vi "SPI_Project.vi"() -> ()   [LabVIEW 2019]
uses:
  <vilib>/rvi/eio/common/nirviEmuTemplateMethod_errors.vi
  <vilib>/eio/EIONode/EIONode.xnode
  <vilib>/eio/EIOMethodNode/EIOMethodNode.xnode
panel:
  out "Device":u32
  in  "Dummy":u8 format="%b"
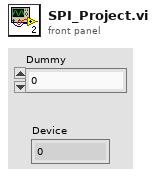
[diagram p1: front panel]
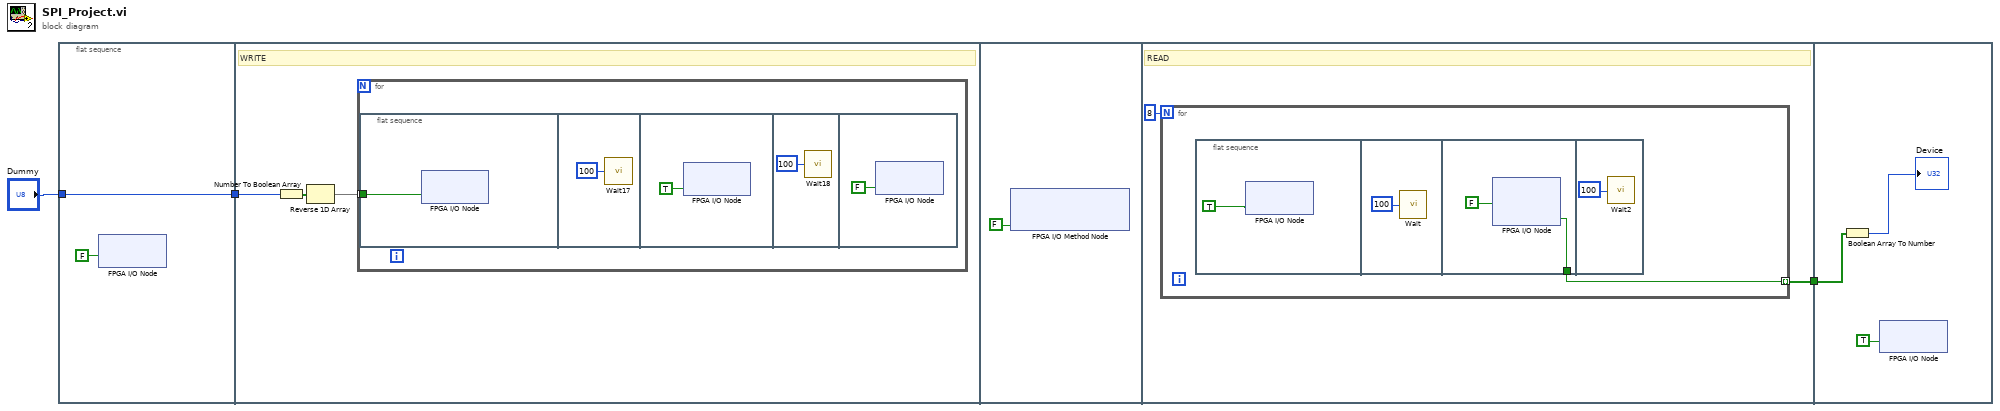
[diagram p0: block diagram]
diagram:
  n1 = flat-sequence {
    tunnel: "Dummy" -> [w5]
    tunnel: [w5] -> w2
    tunnel: w2 -> [w7]
    tunnel: [w16] -> w1
    tunnel: w1 -> [w24]
    frame #0 {
      n2 = xnode "FPGA I/O Node"("CS"=FALSE ("ConnectorB/DIO4")) -> ()  [unwired: 1 in, 1 out]
    }
    frame #1 {
      # "WRITE"
      n3 = Number To Boolean Array(number=w7) -> (Boolean array=w8:bool[])
      n4 = Reverse 1D Array(array=w8) -> (reversed array=w6:bool[])
      n5 = for {
        tunnel: w6 -> [w9] mode=indexing
        n6 = flat-sequence {
          tunnel: w9 -> [w10]
          frame #0 {
            n7 = xnode "FPGA I/O Node"("SDA"=w10) -> ()  [unwired: 1 in, 1 out]
          }
          frame #1 {
            n8 = call "Wait17"("Count(Ticks)"=u32 100) -> ()  [unwired: 1 out]
          }
          frame #2 {
            n9 = xnode "FPGA I/O Node"("SCL"=TRUE ("ConnectorB/DIO0")) -> ()  [unwired: 1 in, 1 out]
          }
          frame #3 {
            n10 = call "Wait18"("Count(Ticks)"=u32 100) -> ()  [unwired: 1 out]
          }
          frame #4 {
            n11 = xnode "FPGA I/O Node"("SCL"=FALSE ("ConnectorB/DIO0")) -> ()  [unwired: 1 in, 1 out]
          }
        }
      }
    }
    frame #2 {
      n12 = xnode "FPGA I/O Method Node"("Enable"=FALSE) -> ()  [unwired: 1 in, 1 out]
    }
    frame #3 {
      # "READ"
      n13 = for {
        N: 8 -> [_]
        tunnel: [w18] -> w16 mode=indexing
        n14 = flat-sequence {
          tunnel: [w21] -> w18
          frame #0 {
            n15 = xnode "FPGA I/O Node"("SCL"=TRUE ("ConnectorB/DIO0")) -> ()  [unwired: 1 in, 1 out]
          }
          frame #1 {
            n16 = call "Wait"("Count(Ticks)"=u32 100) -> ()  [unwired: 1 out]
          }
          frame #2 {
            n17 = xnode "FPGA I/O Node"("SCL"=FALSE ("ConnectorB/DIO0")) -> ("SDA"=w21:bool)  [unwired: 2 in, 2 out]
          }
          frame #3 {
            n18 = call "Wait2"("Count(Ticks)"=u32 100) -> ()  [unwired: 1 out]
          }
        }
      }
    }
    frame #4 {
      n19 = Boolean Array To Number(Boolean array=w24) -> (number=→"Device":u8)
      n20 = xnode "FPGA I/O Node"("CS"=TRUE ("ConnectorB/DIO4")) -> ()  [unwired: 1 in, 1 out]
    }
  }
